vi "nanocal -- nuclear schottky fit V8.vi"() -> ()   [LabVIEW 2021] (continued)
\"Reoff\" -> 0.000000000000   ,  \"Imoff\" -> 0.000000000000   ,  \"στ1\" -> 0.000000000000   ,  \"στS\" -> 0.000000000000   ,  \"στN\" -> 0.000000000000   ,  \"τ11 \" -> 0.000000000000   ,  \"τ12\" -> 0.000000000000   ,  \"τ22\" -> 0.000000000000   ,  \"τN1\" -> 0.000000000000   ,  \"τN2\" -> 0.000000000000   ,  \"σηlogτ1 \" -> 0.000000000000   ,  \"σηlogτS\" -> 0.000000000000   ,  \"σηlogτN\" -> 0.000000000000   ,  \"σlogτ1\" -> 0.000000000000   ,  \"σlogτS\" -> 0.000000000000   ,  \"σlogτN\" -> 0.000000000000   ,  \"σητ1\" -> 0.000000000000   ,  \"σητS \" -> 0.000000000000   ,  \"σητN\" -> 0.000000000000    |>   , \n\"IDS0616_220610_RAW_cal__ref_\" ->   <|    \"ζ\" -> 0.021580744060   ,  \"τ1\" -> 0.018863304594   ,  \"τS\" -> 0.006040479317   ,  \"τN\" -> 0.000001032935   ,  \"τC\" -> 0.001981910818   ,  \"κ0\" -> 0.000000054950   ,  \"mm1\" -> 0.000031813825   ,  \"mm2\" -> 0.008120137752   ,  \"mm3\" -> 0.018865156416   ,  \"T\" -> 5.700000000000   ,  \"B\" -> 5.000000000000   ,  \"θ\" -> 90.000000000000   ,  \"Reoff\" -> 0.000000000000   ,  \"Imoff\" -> 0.000000000000   ,  \"στ1\" -> 0.086753021410   ,  \"στS\" -> 0.000000692284   ,  \"στN\" -> 0.000003593763   ,  \"τ11 \" -> 0.000000000000   ,  \"τ12\" -> 0.000000000000   ,  \"τ22\" -> 0.000000000000   ,  \"τN1\" -> 0.000000000000   ,  \"τN2\" -> 0.000000000000   ,  \"σηlogτ1 \" -> 0.078147370775   ,  \"σηlogτS\" -> 0.000000144573   ,  \"σηlogτN\" -> 0.120525182848   ,  \"σlogτ1\" -> 4.599036238749   ,  \"σlogτS\" -> 0.000114607395   ,  \"σlogτN\" -> 3.479176616069   ,  \"σητ1\" -> 0.001474117658   ,  \"σητS \" -> 0.000000000873   ,  \"σητN\" -> 0.000000124495    |>   , \n\"IDS0616_220610_RAW_cal__sam_\" ->   <|    \"ζ\" -> 0.000000000000   ,  \"τ1\" -> 0.000000000000   ,  \"τS\" -> 0.000000000000   ,  \"τN\" -> 0.000000000000   ,  \"τC\" -> 0.000000000000   ,  \"κ0\" -> 0.000000000000   ,  \"mm1\" -> 0.000000000000   ,  \"mm2\" -> 0.000000000000   ,  \"mm3\" -> 0.000000000000   ,  \"T\" -> 5.700000000000   ,  \"B\" -> 5.000000000000   ,  \"θ\" -> 90.000000000000   ,  \"Reoff\" -> 0.000000000000   ,  \"Imoff\" -> 0.000000000000   ,  \"στ1\" -> 0.000000000000   ,  \"στS\" -> 0.000000000000   ,  \"στN\" -> 0.000000000000   ,  \"τ11 \" -> 0.000000000000   ,  \"τ12\" -> 0.000000000000   ,  \"τ22\" -> 0.000000000000   ,  \"τN1\" -> 0.000000000000   ,  \"τN2\" -> 0.000000000000   ,  \"σηlogτ1 \" -> 0.000000000000   ,  \"σηlogτS\" -> 0.000000000000   ,  \"σηlogτN\" -> 0.000000000000   ,  \"σlogτ1\" -> 0.000000000000   ,  \"σlogτS\" -> 0.000000000000   ,  \"σlogτN\" -> 0.000000000000   ,  \"σητ1\" -> 0.000000000000   ,  \"σητS \" -> 0.000000000000   ,  \"σητN\" -> 0.000000000000    |>   , \n\"IDS0618_220610_RAW_cal__ref_\" ->   <|    \"ζ\" -> 0.037056549880   ,  \"τ1\" -> 0.018725402068   ,  \"τS\" -> 0.027332501190   ,  \"τN\" -> 0.000869050800   ,  \"τC\" -> 0.001924166709   ,  \"κ0\" -> 0.000000003749   ,  \"mm1\" -> 0.000064521634   ,  \"mm2\" -> 0.017486567655   ,  \"mm3\" -> 0.032345083697   ,  \"T\" -> 0.620000000000   ,  \"B\" -> 8.000000000000   ,  \"θ\" -> 90.000000000000   ,  \"Reoff\" -> 0.000000000000   ,  \"Imoff\" -> 0.000000000000   ,  \"στ1\" -> 0.000271617546   ,  \"στS\" -> 0.000004778676   ,  \"στN\" -> 0.000006417045   ,  \"τ11 \" -> 0.000000000000   ,  \"τ12\" -> 0.000000000000   ,  \"τ22\" -> 0.000000000000   ,  \"τN1\" -> 0.000000000000   ,  \"τN2\" -> 0.000000000000   ,  \"σηlogτ1 \" -> 0.143200048871   ,  \"σηlogτS\" -> 0.000251046394   ,  \"σηlogτN\" -> 0.135387426751   ,  \"σlogτ1\" -> 0.014505298451   ,  \"σlogτS\" -> 0.000174834918   ,  \"σlogτN\" -> 0.007383969732   ,  \"σητ1\" -> 0.002681478491   ,  \"σητS \" -> 0.000006861726   ,  \"σητN\" -> 0.000117658552    |>   , \n\"IDS0618_220610_RAW_cal__sam_\" ->   <|    \"ζ\" -> 0.000000000000   ,  \"τ1\" -> 0.000000000000   ,  \"τS\" -> 0.000000000000   ,  \"τN\" -> 0.000000000000   ,  \"τC\" -> 0.000000000000   ,  \"κ0\" -> 0.000000000000   ,  \"mm1\" -> 0.000000000000   ,  \"mm2\" -> 0.000000000000   ,  \"mm3\" -> 0.000000000000   ,  \"T\" -> 0.620000000000   ,  \"B\" -> 8.000000000000   ,  \"θ\" -> 90.000000000000   ,  \"Reoff\" -> 0.000000000000   ,  \"Imoff\" -> 0.000000000000   ,  \"στ1\" -> 0.000000000000   ,  \"στS\" -> 0.000000000000   ,  \"στN\" -> 0.000000000000   ,  \"τ11 \" -> 0.000000000000   ,  \"τ12\" -> 0.000000000000   ,  \"τ22\" -> 0.000000000000   ,  \"τN1\" -> 0.000000000000   ,  \"τN2\" -> 0.000000000000   ,  \"σηlogτ1 \" -> 0.000000000000   ,  \"σηlogτS\" -> 0.000000000000   ,  \"σηlogτN\" -> 0.000000000000   ,  \"σlogτ1\" -> 0.000000000000   ,  \"σlogτS\" -> 0.000000000000   ,  \"σlogτN\" -> 0.000000000000   ,  \"σητ1\" -> 0.000000000000   ,  \"σητS \" -> 0.000000000000   ,  \"σητN\" -> 0.000000000000    |>   , \n\"IDS0619_220610_RAW_cal__ref_\" ->   <|    \"ζ\" -> 0.022285334240   ,  \"τ1\" -> 0.023690071245   ,  \"τS\" -> 0.019354849977   ,  \"τN\" -> 0.000243089691   ,  \"τC\" -> 0.002524640152   ,  \"κ0\" -> 0.000000007189   ,  \"mm1\" -> 0.000048915318   ,  \"mm2\" -> 0.020603538471   ,  \"mm3\" -> 0.025596943911   ,  \"T\" -> 1.120000000000   ,  \"B\" -> 8.000000000000   ,  \"θ\" -> 90.000000000000   ,  \"Reoff\" -> 0.000000000000   ,  \"Imoff\" -> 0.000000000000   ,  \"στ1\" -> 0.000555160768   ,  \"στS\" -> 0.000001577745   ,  \"στN\" -> 0.000003357454   ,  \"τ11 \" -> 0.000000000000   ,  \"τ12\" -> 0.000000000000   ,  \"τ22\" -> 0.000000000000   ,  \"τN1\" -> 0.000000000000   ,  \"τN2\" -> 0.000000000000   ,  \"σηlogτ1 \" -> 0.107205120132   ,  \"σηlogτS\" -> 0.000041987587   ,  \"σηlogτN\" -> 0.127923521319   ,  \"σlogτ1\" -> 0.023434322442   ,  \"σlogτS\" -> 0.000081516797   ,  \"σlogτN\" -> 0.013811587104   ,  \"σητ1\" -> 0.002539696934   ,  \"σητS \" -> 0.000000812663   ,  \"σητN\" -> 0.000031096889    |>   , \n\"IDS0619_220610_RAW_cal__sam_\" ->   <|    \"ζ\" -> 0.000000000000   ,  \"τ1\" -> 0.000000000000   ,  \"τS\" -> 0.000000000000   ,  \"τN\" -> 0.000000000000   ,  \"τC\" -> 0.000000000000   ,  \"κ0\" -> 0.000000000000   ,  \"mm1\" -> 0.000000000000   ,  \"mm2\" -> 0.000000000000   ,  \"mm3\" -> 0.000000000000   ,  \"T\" -> 1.120000000000   ,  \"B\" -> 8.000000000000   ,  \"θ\" -> 90.000000000000   ,  \"Reoff\" -> 0.000000000000   ,  \"Imoff\" -> 0.000000000000   ,  \"στ1\" -> 0.000000000000   ,  \"στS\" -> 0.000000000000   ,  \"στN\" -> 0.000000000000   ,  \"τ11 \" -> 0.000000000000   ,  \"τ12\" -> 0.000000000000   ,  \"τ22\" -> 0.000000000000   ,  \"τN1\" -> 0.000000000000   ,  \"τN2\" -> 0.000000000000   ,  \"σηlogτ1 \" -> 0.000000000000   ,  \"σηlogτS\" -> 0.000000000000   ,  \"σηlogτN\" -> 0.000000000000   ,  \"σlogτ1\" -> 0.000000000000   ,  \"σlogτS\" -> 0.000000000000   ,  \"σlogτN\" -> 0.000000000000   ,  \"σητ1\" -> 0.000000000000   ,  \"σητS \" -> 0.000000000000   ,  \"σητN\" -> 0.000000000000    |>   , \n\"IDS0620_220610_RAW_cal__ref_\" ->   <|    \"ζ\" -> 0.017708509932   ,  \"τ1\" -> 0.018998736540   ,  \"τS\" -> 0.013522892780   ,  \"τN\" -> 0.000028025441   ,  \"τC\" -> 0.002986591079   ,  \"κ0\" -> 0.000000012545   ,  \"mm1\" -> 0.000042810551   ,  \"mm2\" -> 0.016516471437   ,  \"mm3\" -> 0.019216930422   ,  \"T\" -> 1.900000000000   ,  \"B\" -> 8.000000000000   ,  \"θ\" -> 90.000000000000   ,  \"Reoff\" -> -322448.979591836221   ,  \"Imoff\" -> 0.000000000000   ,  \"στ1\" -> 0.140264404305   ,  \"στS\" -> 0.000129912637   ,  \"στN\" -> 0.061579435163   ,  \"τ11 \" -> 0.000000000000   ,  \"τ12\" -> 0.000000000000   ,  \"τ22\" -> 0.000000000000   ,  \"τN1\" -> 0.000000000000   ,  \"τN2\" -> 0.000000000000   ,  \"σηlogτ1 \" -> 0.000000000000   ,  \"σηlogτS\" -> 0.000000000000   ,  \"σηlogτN\" -> 0.000000000000   ,  \"σlogτ1\" -> 0.000000000000   ,  \"σlogτS\" -> 0.000000000000   ,  \"σlogτN\" -> 0.000000000000   ,  \"σητ1\" -> 0.000000000000   ,  \"σητS \" -> 0.000000000000   ,  \"σητN\" -> 0.000000000000    |>   , \n\"IDS0620_220610_RAW_cal__sam_\" ->   <|    \"ζ\" -> 0.000000000000   ,  \"τ1\" -> 0.000000000000   ,  \"τS\" -> 0.000000000000   ,  \"τN\" -> 0.000000000000   ,  \"τC\" -> 0.000000000000   ,  \"κ0\" -> 0.000000000000   ,  \"mm1\" -> 0.000000000000   ,  \"mm2\" -> 0.000000000000   ,  \"mm3\" -> 0.000000000000   ,  \"T\" -> 1.900000000000   ,  \"B\" -> 8.000000000000   ,  \"θ\" -> 90.000000000000   ,  \"Reoff\" -> 0.000000000000   ,  \"Imoff\" -> 0.000000000000   ,  \"στ1\" -> 0.000000000000   ,  \"στS\" -> 0.000000000000   ,  \"στN\" -> 0.000000000000   ,  \"τ11 \" -> 0.000000000000   ,  \"τ12\" -> 0.000000000000   ,  \"τ22\" -> 0.000000000000   ,  \"τN1\" -> 0.000000000000   ,  \"τN2\" -> 0.000000000000   ,  \"σηlogτ1 \" -> 0.000000000000   ,  \"σηlogτS\" -> 0.000000000000   ,  \"σηlogτN\" -> 0.000000000000   ,  \"σlogτ1\" -> 0.000000000000   ,  \"σlogτS\" -> 0.000000000000   ,  \"σlogτN\" -> 0.000000000000   ,  \"σητ1\" -> 0.000000000000   ,  \"σητS \" -> 0.000000000000   ,  \"σητN\" -> 0.000000000000    |>   , \n\"IDS0621_220610_RAW_cal__ref_\" ->   <|    \"ζ\" -> 0.017222795450   ,  \"τ1\" -> 0.018997433498   ,  \"τS\" -> 0.009525458339   ,  \"τN\" -> 0.000004659714   ,  \"τC\" -> 0.002829107724   ,  \"κ0\" -> 0.000000022378   ,  \"mm1\" -> 0.000037185565   ,  \"mm2\" -> 0.012472383052   ,  \"mm3\" -> 0.019011225932   ,  \"T\" -> 3.100000000000   ,  \"B\" -> 8.000000000000   ,  \"θ\" -> 90.000000000000   ,  \"Reoff\" -> -175510.204081632662   ,  \"Imoff\" -> 0.000000000000   ,  \"στ1\" -> 1.184463822187   ,  \"στS\" -> 0.000211196697   ,  \"στN\" -> 0.576926670035   ,  \"τ11 \" -> 0.000000000000   ,  \"τ12\" -> 0.000000000000   ,  \"τ22\" -> 0.000000000000   ,  \"τN1\" -> 0.000000000000   ,  \"τN2\" -> 0.000000000000   ,  \"σηlogτ1 \" -> 0.000000000000   ,  \"σηlogτS\" -> 0.000000000000   ,  \"σηlogτN\" -> 0.000000000000   ,  \"σlogτ1\" -> 0.000000000000   ,  \"σlogτS\" -> 0.000000000000   ,  \"σlogτN\" -> 0.000000000000   ,  \"σητ1\" -> 0.000000000000   ,  \"σητS \" -> 0.000000000000   ,  \"σητN\" -> 0.000000000000    |>   , \n\"IDS0621_220610_RAW_cal__sam_\" ->   <|    \"ζ\" -> 0.000000000000   ,  \"τ1\" -> 0.000000000000   ,  \"τS\" -> 0.000000000000   ,  \"τN\" -> 0.000000000000   ,  \"τC\" -> 0.000000000000   ,  \"κ0\" -> 0.000000000000   ,  \"mm1\" -> 0.000000000000   ,  \"mm2\" -> 0.000000000000   ,  \"mm3\" -> 0.000000000000   ,  \"T\" -> 3.100000000000   ,  \"B\" -> 8.000000000000   ,  \"θ\" -> 90.000000000000   ,  \"Reoff\" -> 0.000000000000   ,  \"Imoff\" -> 0.000000000000   ,  \"στ1\" -> 0.000000000000   ,  \"στS\" -> 0.000000000000   ,  \"στN\" -> 0.000000000000   ,  \"τ11 \" -> 0.000000000000   ,  \"τ12\" -> 0.000000000000   ,  \"τ22\" -> 0.000000000000   ,  \"τN1\" -> 0.000000000000   ,  \"τN2\" -> 0.000000000000   ,  \"σηlogτ1 \" -> 0.000000000000   ,  \"σηlogτS\" -> 0.000000000000   ,  \"σηlogτN\" -> 0.000000000000   ,  \"σlogτ1\" -> 0.000000000000   ,  \"σlogτS\" -> 0.000000000000   ,  \"σlogτN\" -> 0.000000000000   ,  \"σητ1\" -> 0.000000000000   ,  \"σητS \" -> 0.000000000000   ,  \"σητN\" -> 0.000000000000    |>   , \n\"IDS0622_220610_RAW_cal__ref_\" ->   <|    \"ζ\" -> 0.018802685442   ,  \"τ1\" -> 0.018950322094   ,  \"τS\" -> 0.005932159284   ,  \"τN\" -> 0.000000659524   ,  \"τC\" -> 0.002206206702   ,  \"κ0\" -> 0.000000055128   ,  \"mm1\" -> 0.000029937026   ,  \"mm2\" -> 0.008219455491   ,  \"mm3\" -> 0.018951508013   ,  \"T\" -> 5.700000000000   ,  \"B\" -> 8.000000000000   ,  \"θ\" -> 90.000000000000   ,  \"Reoff\" -> -102040.816326530650   ,  \"Imoff\" -> 0.000000000000   ,  \"στ1\" -> 16.146666898973   ,  \"στS\" -> 0.000465319371   ,  \"στN\" -> 9.721658755114   ,  \"τ11 \" -> 0.000000000000   ,  \"τ12\" -> 0.000000000000   ,  \"τ22\" -> 0.000000000000   ,  \"τN1\" -> 0.000000000000   ,  \"τN2\" -> 0.000000000000   ,  \"σηlogτ1 \" -> 0.000000000000   ,  \"σηlogτS\" -> 0.000000000000   ,  \"σηlogτN\" -> 0.000000000000   ,  \"σlogτ1\" -> 0.000000000000   ,  \"σlogτS\" -> 0.000000000000   ,  \"σlogτN\" -> 0.000000000000   ,  \"σητ1\" -> 0.000000000000   ,  \"σητS \" -> 0.000000000000   ,  \"σητN\" -> 0.000000000000    |>   , \n\"IDS0622_220610_RAW_cal__sam_\" ->   <|    \"ζ\" -> 0.000000000000   ,  \"τ1\" -> 0.000000000000   ,  \"τS\" -> 0.000000000000   ,  \"τN\" -> 0.000000000000   ,  \"τC\" -> 0.000000000000   ,  \"κ0\" -> 0.000000000000   ,  \"mm1\" -> 0.000000000000   ,  \"mm2\" -> 0.000000000000   ,  \"mm3\" -> 0.000000000000   ,  \"T\" -> 5.700000000000   ,  \"B\" -> 8.000000000000   ,  \"θ\" -> 90.000000000000   ,  \"Reoff\" -> 0.000000000000   ,  \"Imoff\" -> 0.000000000000   ,  \"στ1\" -> 0.000000000000   ,  \"στS\" -> 0.000000000000   ,  \"στN\" -> 0.000000000000   ,  \"τ11 \" -> 0.000000000000   ,  \"τ12\" -> 0.000000000000   ,  \"τ22\" -> 0.000000000000   ,  \"τN1\" -> 0.000000000000   ,  \"τN2\" -> 0.000000000000   ,  \"σηlogτ1 \" -> 0.000000000000   ,  \"σηlogτS\" -> 0.000000000000   ,  \"σηlogτN\" -> 0.000000000000   ,  \"σlogτ1\" -> 0.000000000000   ,  \"σlogτS\" -> 0.000000000000   ,  \"σlogτN\" -> 0.000000000000   ,  \"σητ1\" -> 0.000000000000   ,  \"σητS \" -> 0.000000000000   ,  \"σητN\" -> 0.000000000000    |>   , \n\"IDS0624_220611_RAW_cal__ref_\" ->   <|    \"ζ\" -> 0.236945855383   ,  \"τ1\" -> 0.047928938722   ,  \"τS\" -> 0.040227228605   ,  \"τN\" -> 0.063271724608   ,  \"τC\" -> 0.000912127152   ,  \"κ0\" -> 0.000000000938   ,  \"mm1\" -> 0.000172149820   ,  \"mm2\" -> 0.014967198661   ,  \"mm3\" -> 0.161724318607   ,  \"T\" -> 0.200000000000   ,  \"B\" -> 10.000000000000   ,  \"θ\" -> 90.000000000000   ,  \"Reoff\" -> 0.000000000000   ,  \"Imoff\" -> 0.000000000000   ,  \"στ1\" -> 0.000044813488   ,  \"στS\" -> 0.000011433304   ,  \"στN\" -> 0.000038242973   ,  \"τ11 \" -> 0.000000000000   ,  \"τ12\" -> 0.000000000000   ,  \"τ22\" -> 0.000000000000   ,  \"τN1\" -> 0.000000000000   ,  \"τN2\" -> 0.000000000000   ,  \"σηlogτ1 \" -> 0.116274669687   ,  \"σηlogτS\" -> 0.004088772446   ,  \"σηlogτN\" -> 0.139680235023   ,  \"σlogτ1\" -> 0.000934998552   ,  \"σlogτS\" -> 0.000284218031   ,  \"σlogτN\" -> 0.000604424386   ,  \"σητ1\" -> 0.005572921518   ,  \"σητS \" -> 0.000164479984   ,  \"σητN\" -> 0.008837809363    |>   , \n\"IDS0624_220611_RAW_cal__sam_\" ->   <|    \"ζ\" -> 0.000000000000   ,  \"τ1\" -> 0.000000000000   ,  \"τS\" -> 0.000000000000   ,  \"τN\" -> 0.000000000000   ,  \"τC\" -> 0.000000000000   ,  \"κ0\" -> 0.000000000000   ,  \"mm1\" -> 0.000000000000   ,  \"mm2\" -> 0.000000000000   ,  \"mm3\" -> 0.000000000000   ,  \"T\" -> 0.200000000000   ,  \"B\" -> 10.000000000000   ,  \"θ\" -> 90.000000000000   ,  \"Reoff\" -> 0.000000000000   ,  \"Imoff\" -> 0.000000000000   ,  \"στ1\" -> 0.000000000000   ,  \"στS\" -> 0.000000000000   ,  \"στN\" -> 0.000000000000   ,  \"τ11 \" -> 0.000000000000   ,  \"τ12\" -> 0.000000000000   ,  \"τ22\" -> 0.000000000000   ,  \"τN1\" -> 0.000000000000   ,  \"τN2\" -> 0.000000000000   ,  \"σηlogτ1 \" -> 0.000000000000   ,  \"σηlogτS\" -> 0.000000000000   ,  \"σηlogτN\" -> 0.000000000000   ,  \"σlogτ1\" -> 0.000000000000   ,  \"σlogτS\" -> 0.000000000000   ,  \"σlogτN\" -> 0.000000000000   ,  \"σητ1\" -> 0.000000000000   ,  \"σητS \" -> 0.000000000000   ,  \"σητN\" -> 0.000000000000    |>   , \n\"IDS0625_220611_RAW_cal__ref_\" ->   <|    \"ζ\" -> 0.327025562837   ,  \"τ1\" -> 0.059339000703   ,  \"τS\" -> 0.049734125673   ,  \"τN\" -> 0.113807285584   ,  \"τC\" -> 0.000851803177   ,  \"κ0\" -> 0.000000000764   ,  \"mm1\" -> 0.000207869539   ,  \"mm2\" -> 0.015100054741   ,  \"mm3\" -> 0.261906512920   ,  \"T\" -> 0.170000000000   ,  \"B\" -> 10.000000000000   ,  \"θ\" -> 90.000000000000   ,  \"Reoff\" -> 0.000000000000   ,  \"Imoff\" -> 0.000000000000   ,  \"στ1\" -> 0.000104711962   ,  \"στS\" -> 0.000034023066   ,  \"στN\" -> 0.000130609835   ,  \"τ11 \" -> 0.000000000000   ,  \"τ12\" -> 0.000000000000   ,  \"τ22\" -> 0.000000000000   ,  \"τN1\" -> 0.000000000000   ,  \"τN2\" -> 0.000000000000   ,  \"σηlogτ1 \" -> 0.122338501744   ,  \"σηlogτS\" -> 0.005402997656   ,  \"σηlogτN\" -> 0.146638117575   ,  \"σlogτ1\" -> 0.001764639795   ,  \"σlogτS\" -> 0.000684099005   ,  \"σlogτN\" -> 0.001147640370   ,  \"σητ1\" -> 0.007259444441   ,  \"σητS \" -> 0.000268713364   ,  \"σητN\" -> 0.016688486124    |>   , \n\"IDS0625_220611_RAW_cal__sam_\" ->   <|    \"ζ\" -> 0.000000000000   ,  \"τ1\" -> 0.000000000000   ,  \"τS\" -> 0.000000000000   ,  \"τN\" -> 0.000000000000   ,  \"τC\" -> 0.000000000000   ,  \"κ0\" -> 0.000000000000   ,  \"mm1\" -> 0.000000000000   ,  \"mm2\" -> 0.000000000000   ,  \"mm3\" -> 0.000000000000   ,  \"T\" -> 0.170000000000   ,  \"B\" -> 10.000000000000   ,  \"θ\" -> 90.000000000000   ,  \"Reoff\" -> 0.000000000000   ,  \"Imoff\" -> 0.000000000000   ,  \"στ1\" -> 0.000000000000   ,  \"στS\" -> 0.000000000000   ,  \"στN\" -> 0.000000000000   ,  \"τ11 \" -> 0.000000000000   ,  \"τ12\" -> 0.000000000000   ,  \"τ22\" -> 0.000000000000   ,  \"τN1\" -> 0.000000000000   ,  \"τN2\" -> 0.000000000000   ,  \"σηlogτ1 \" -> 0.000000000000   ,  \"σηlogτS\" -> 0.000000000000   ,  \"σηlogτN\" -> 0.000000000000   ,  \"σlogτ1\" -> 0.000000000000   ,  \"σlogτS\" -> 0.000000000000   ,  \"σlogτN\" -> 0.000000000000   ,  \"σητ1\" -> 0.000000000000   ,  \"σητS \" -> 0.000000000000   ,  \"σητN\" -> 0.000000000000    |>   , \n\"IDS0626_220611_RAW_cal__ref_\" ->   <|    \"ζ\" -> 0.413398104897   ,  \"τ1\" -> 0.067875745841   ,  \"τS\" -> 0.063032069928   ,  \"τN\" -> 0.190750500145   ,  \"τC\" -> 0.000838943281   ,  \"κ0\" -> 0.000000000639   ,  \"mm1\" -> 0.000243732197   ,  \"mm2\" -> 0.014761841095   ,  \"mm3\" -> 0.412404919429   ,  \"T\" -> 0.150000000000   ,  \"B\" -> 10.000000000000   ,  \"θ\" -> 90.000000000000   ,  \"Reoff\" -> 0.000000000000   ,  \"Imoff\" -> 0.000000000000   ,  \"στ1\" -> 0.000192212133   ,  \"στS\" -> 0.000084399120   ,  \"στN\" -> 0.000341477666   ,  \"τ11 \" -> 0.000000000000   ,  \"τ12\" -> 0.000000000000   ,  \"τ22\" -> 0.000000000000   ,  \"τN1\" -> 0.000000000000   ,  \"τN2\" -> 0.000000000000   ,  \"σηlogτ1 \" -> 0.134243827848   ,  \"σηlogτS\" -> 0.007146311807   ,  \"σηlogτN\" -> 0.157301214691   ,  \"σlogτ1\" -> 0.002831823508   ,  \"σlogτS\" -> 0.001338986966   ,  \"σlogτN\" -> 0.001790179662   ,  \"σητ1\" -> 0.009111899940   ,  \"σητS \" -> 0.000450446826   ,  \"σητN\" -> 0.030005285376    |>   , \n\"IDS0626_220611_RAW_cal__sam_\" ->   <|    \"ζ\" -> 0.000000000000   ,  \"τ1\" -> 0.000000000000   ,  \"τS\" -> 0.000000000000   ,  \"τN\" -> 0.000000000000   ,  \"τC\" -> 0.000000000000   ,  \"κ0\" -> 0.000000000000   ,  \"mm1\" -> 0.000000000000   ,  \"mm2\" -> 0.000000000000   ,  \"mm3\" -> 0.000000000000   ,  \"T\" -> 0.150000000000   ,  \"B\" -> 10.000000000000   ,  \"θ\" -> 90.000000000000   ,  \"Reoff\" -> 0.000000000000   ,  \"Imoff\" -> 0.000000000000   ,  \"στ1\" -> 0.000000000000   ,  \"στS\" -> 0.000000000000   ,  \"στN\" -> 0.000000000000   ,  \"τ11 \" -> 0.000000000000   ,  \"τ12\" -> 0.000000000000   ,  \"τ22\" -> 0.000000000000   ,  \"τN1\" -> 0.000000000000   ,  \"τN2\" -> 0.000000000000   ,  \"σηlogτ1 \" -> 0.000000000000   ,  \"σηlogτS\" -> 0.000000000000   ,  \"σηlogτN\" -> 0.000000000000   ,  \"σlogτ1\" -> 0.000000000000   ,  \"σlogτS\" -> 0.000000000000   ,  \"σlogτN\" -> 0.000000000000   ,  \"σητ1\" -> 0.000000000000   ,  \"σητS \" -> 0.000000000000   ,  \"σητN\" -> 0.000000000000    |>   , \n\"IDS0627_220611_RAW_cal__ref_\" ->   <|    \"ζ\" -> 0.627345868591   ,  \"τ1\" -> 0.082512030624   ,  \"τS\" -> 0.111539942988   ,  \"τN\" -> 0.459820261039   ,  \"τC\" -> 0.000856922343   ,  \"κ0\" -> 0.000000000480   ,  \"mm1\" -> 0.000329372323   ,  \"mm2\" -> 0.015054692399   ,  \"mm3\" -> 0.997785555745   ,  \"T\" -> 0.120000000000   ,  \"B\" -> 10.000000000000   ,  \"θ\" -> 90.000000000000   ,  \"Reoff\" -> 0.000000000000   ,  \"Imoff\" -> 0.000000000000   ,  \"στ1\" -> 0.000378111787   ,  \"στS\" -> 0.000316880051   ,  \"στN\" -> 0.001160403216   ,  \"τ11 \" -> 0.000000000000   ,  \"τ12\" -> 0.000000000000   ,  \"τ22\" -> 0.000000000000   ,  \"τN1\" -> 0.000000000000   ,  \"τN2\" -> 0.000000000000   ,  \"σηlogτ1 \" -> 0.166706810062   ,  \"σηlogτS\" -> 0.011257222829   ,  \"σηlogτN\" -> 0.184131010310   ,  \"σlogτ1\" -> 0.004582504926   ,  \"σlogτS\" -> 0.002840955825   ,  \"σlogτN\" -> 0.002523601752   ,  \"σητ1\" -> 0.013755317417   ,  \"σητS \" -> 0.001255629993   ,  \"σητN\" -> 0.084667169226    |>   , \n\"IDS0627_220611_RAW_cal__sam_\" ->   <|    \"ζ\" -> 0.000000000000   ,  \"τ1\" -> 0.000000000000   ,  \"τS\" -> 0.000000000000   ,  \"τN\" -> 0.000000000000   ,  \"τC\" -> 0.000000000000   ,  \"κ0\" -> 0.000000000000   ,  \"mm1\" -> 0.000000000000   ,  \"mm2\" -> 0.000000000000   ,  \"mm3\" -> 0.000000000000   ,  \"T\" -> 0.120000000000   ,  \"B\" -> 10.000000000000   ,  \"θ\" -> 90.000000000000   ,  \"Reoff\" -> 0.000000000000   ,  \"Imoff\" -> 0.000000000000   ,  \"στ1\" -> 0.000000000000   ,  \"στS\" -> 0.000000000000   ,  \"στN\" -> 0.000000000000   ,  \"τ11 \" -> 0.000000000000   ,  \"τ12\" -> 0.000000000000   ,  \"τ22\" -> 0.000000000000   ,  \"τN1\" -> 0.000000000000   ,  \"τN2\" -> 0.000000000000   ,  \"σηlogτ1 \" -> 0.000000000000   ,  \"σηlogτS\" -> 0.000000000000   ,  \"σηlogτN\" -> 0.000000000000   ,  \"σlogτ1\" -> 0.000000000000   ,  \"σlogτS\" -> 0.000000000000   ,  \"σlogτN\" -> 0.000000000000   ,  \"σητ1\" -> 0.000000000000   ,  \"σητS \" -> 0.000000000000   ,  \"σητN\" -> 0.000000000000    |>   , \n\"IDS0628_220611_RAW_cal__ref_\" ->   <|    \"ζ\" -> 0.152770220737   ,  \"τ1\" -> 0.036198364925   ,  \"τS\" -> 0.033549808091   ,  \"τN\" -> 0.027206802922   ,  \"τC\" -> 0.001036197063   ,  \"κ0\" -> 0.000000001265   ,  \"mm1\" -> 0.000134182447   ,  \"mm2\" -> 0.015662270095   ,  \"mm3\" -> 0.091476521334   ,  \"T\" -> 0.250000000000   ,  \"B\" -> 10.000000000000   ,  \"θ\" -> 90.000000000000   ,  \"Reoff\" -> 0.000000000000   ,  \"Imoff\" -> 0.000000000000   ,  \"στ1\" -> 0.000013390131   ,  \"στS\" -> 0.000002421606   ,  \"στN\" -> 0.000006177026   ,  \"τ11 \" -> 0.000000000000   ,  \"τ12\" -> 0.000000000000   ,  \"τ22\" -> 0.000000000000   ,  \"τN1\" -> 0.000000000000   ,  \"τN2\" -> 0.000000000000   ,  \"σηlogτ1 \" -> 0.116147333813   ,  \"σηlogτS\" -> 0.002721053400   ,  \"σηlogτN\" -> 0.134955883548   ,  \"σlogτ1\" -> 0.000369909834   ,  \"σlogτS\" -> 0.000072179437   ,  \"σlogτN\" -> 0.000227039759   ,  \"σητ1\" -> 0.004204343574   ,  \"σητS \" -> 0.000091290819   ,  \"σητN\" -> 0.003671718127    |>   , \n\"IDS0628_220611_RAW_cal__sam_\" ->   <|    \"ζ\" -> 0.000000000000   ,  \"τ1\" -> 0.000000000000   ,  \"τS\" -> 0.000000000000   ,  \"τN\" -> 0.000000000000   ,  \"τC\" -> 0.000000000000   ,  \"κ0\" -> 0.000000000000   ,  \"mm1\" -> 0.000000000000   ,  \"mm2\" -> 0.000000000000   ,  \"mm3\" -> 0.000000000000   ,  \"T\" -> 0.250000000000   ,  \"B\" -> 10.000000000000   ,  \"θ\" -> 90.000000000000   ,  \"Reoff\" -> 0.000000000000   ,  \"Imoff\" -> 0.000000000000   ,  \"στ1\" -> 0.000000000000   ,  \"στS\" -> 0.000000000000   ,  \"στN\" -> 0.000000000000   ,  \"τ11 \" -> 0.000000000000   ,  \"τ12\" -> 0.000000000000   ,  \"τ22\" -> 0.000000000000   ,  \"τN1\" -> 0.000000000000   ,  \"τN2\" -> 0.000000000000   ,  \"σηlogτ1 \" -> 0.000000000000   ,  \"σηlogτS\" -> 0.000000000000   ,  \"σηlogτN\" -> 0.000000000000   ,  \"σlogτ1\" -> 0.000000000000   ,  \"σlogτS\" -> 0.000000000000   ,  \"σlogτN\" -> 0.000000000000   ,  \"σητ1\" -> 0.000000000000   ,  \"σητS \" -> 0.000000000000   ,  \"σητN\" -> 0.000000000000    |>   , \n\"IDS0629_220611_RAW_cal__ref_\" ->   <|    \"ζ\" -> 0.104961058193   ,  \"τ1\" -> 0.030489437824   ,  \"τS\" -> 0.030011872176   ,  \"τN\" -> 0.014021025099   ,  \"τC\" -> 0.001158647608   ,  \"κ0\" -> 0.000000001606   ,  \"mm1\" -> 0.000106671353   ,  \"mm2\" -> 0.016335963882   ,  \"mm3\" -> 0.063860086966   ,  \"T\" -> 0.300000000000   ,  \"B\" -> 10.000000000000   ,  \"θ\" -> 90.000000000000   ,  \"Reoff\" -> 0.000000000000   ,  \"Imoff\" -> 0.000000000000   ,  \"στ1\" -> 0.000007085631   ,  \"στS\" -> 0.000000880275   ,  \"στN\" -> 0.000001925171   ,  \"τ11 \" -> 0.000000000000   ,  \"τ12\" -> 0.000000000000   ,  \"τ22\" -> 0.000000000000   ,  \"τN1\" -> 0.000000000000   ,  \"τN2\" -> 0.000000000000   ,  \"σηlogτ1 \" -> 0.117123612292   ,  \"σηlogτS\" -> 0.001807335056   ,  \"σηlogτN\" -> 0.132991316128   ,  \"σlogτ1\" -> 0.000232396245   ,  \"σlogτS\" -> 0.000029330901   ,  \"σlogτN\" -> 0.000137306042   ,  \"σητ1\" -> 0.003571033095   ,  \"σητS \" -> 0.000054241509   ,  \"σητN\" -> 0.001864674581    |>   , \n\"IDS0629_220611_RAW_cal__sam_\" ->   <|    \"ζ\" -> 0.000000000000   ,  \"τ1\" -> 0.000000000000   ,  \"τS\" -> 0.000000000000   ,  \"τN\" -> 0.000000000000   ,  \"τC\" -> 0.000000000000   ,  \"κ0\" -> 0.000000000000   ,  \"mm1\" -> 0.000000000000   ,  \"mm2\" -> 0.000000000000   ,  \"mm3\" -> 0.000000000000   ,  \"T\" -> 0.300000000000   ,  \"B\" -> 10.000000000000   ,  \"θ\" -> 90.000000000000   ,  \"Reoff\" -> 0.000000000000   ,  \"Imoff\" -> 0.000000000000   ,  \"στ1\" -> 0.000000000000   ,  \"στS\" -> 0.000000000000   ,  \"στN\" -> 0.000000000000   ,  \"τ11 \" -> 0.000000000000   ,  \"τ12\" -> 0.000000000000   ,  \"τ22\" -> 0.000000000000   ,  \"τN1\" -> 0.000000000000   ,  \"τN2\" -> 0.000000000000   ,  \"σηlogτ1 \" -> 0.000000000000   ,  \"σηlogτS\" -> 0.000000000000   ,  \"σηlogτN\" -> 0.000000000000   ,  \"σlogτ1\" -> 0.000000000000   ,  \"σlogτS\" -> 0.000000000000   ,  \"σlogτN\" -> 0.000000000000   ,  \"σητ1\" -> 0.000000000000   ,  \"σητS \" -> 0.000000000000   ,  \"σητN\" -> 0.000000000000    |>   , \n\"IDS0630_220611_RAW_cal__ref_\" ->   <|    \"ζ\" -> 0.075687079530   ,  \"τ1\" -> 0.025692917456   ,  \"τS\" -> 0.027518005635   ,  \"τN\" -> 0.007256477389   ,  \"τC\" -> 0.001413406836   ,  \"κ0\" -> 0.000000002017   ,  \"mm1\" -> 0.000095205662   ,  \"mm2\" -> 0.016621150095   ,  \"mm3\" -> 0.047796430621   ,  \"T\" -> 0.360000000000   ,  \"B\" -> 10.000000000000   ,  \"θ\" -> 90.000000000000   ,  \"Reoff\" -> 0.000000000000   ,  \"Imoff\" -> 0.000000000000   ,  \"στ1\" -> 0.000009211361   ,  \"στS\" -> 0.000000780336   ,  \"στN\" -> 0.000001470575   ,  \"τ11 \" -> 0.000000000000   ,  \"τ12\" -> 0.000000000000   ,  \"τ22\" -> 0.000000000000   ,  \"τN1\" -> 0.000000000000   ,  \"τN2\" -> 0.000000000000   ,  \"σηlogτ1 \" -> 0.121353390675   ,  \"σηlogτS\" -> 0.001216073528   ,  \"σηlogτN\" -> 0.132703139128   ,  \"σlogτ1\" -> 0.000358517508   ,  \"σlogτS\" -> 0.000028357288   ,  \"σlogτN\" -> 0.000202656857   ,  \"σητ1\" -> 0.003117922650   ,  \"σητS \" -> 0.000033463918   ,  \"σητN\" -> 0.000962957328    |>   , \n\"IDS0630_220611_RAW_cal__sam_\" ->   <|    \"ζ\" -> 0.000000000000   ,  \"τ1\" -> 0.000000000000   ,  \"τS\" -> 0.000000000000   ,  \"τN\" -> 0.000000000000   ,  \"τC\" -> 0.000000000000   ,  \"κ0\" -> 0.000000000000   ,  \"mm1\" -> 0.000000000000   ,  \"mm2\" -> 0.000000000000   ,  \"mm3\" -> 0.000000000000   ,  \"T\" -> 0.360000000000   ,  \"B\" -> 10.000000000000   ,  \"θ\" -> 90.000000000000   ,  \"Reoff\" -> 0.000000000000   ,  \"Imoff\" -> 0.000000000000   ,  \"στ1\" -> 0.000000000000   ,  \"στS\" -> 0.000000000000   ,  \"στN\" -> 0.000000000000   ,  \"τ11 \" -> 0.000000000000   ,  \"τ12\" -> 0.000000000000   ,  \"τ22\" -> 0.000000000000   ,  \"τN1\" -> 0.000000000000   ,  \"τN2\" -> 0.000000000000   ,  \"σηlogτ1 \" -> 0.000000000000   ,  \"σηlogτS\" -> 0.000000000000   ,  \"σηlogτN\" -> 0.000000000000   ,  \"σlogτ1\" -> 0.000000000000   ,  \"σlogτS\" -> 0.000000000000   ,  \"σlogτN\" -> 0.000000000000   ,  \"σητ1\" -> 0.000000000000   ,  \"σητS \" -> 0.000000000000   ,  \"σητN\" -> 0.000000000000    |>   , \n\"IDS0631_220611_RAW_cal__ref_\" ->   <|    \"ζ\" -> 0.058935240336   ,  \"τ1\" -> 0.021193518217   ,  \"τS\" -> 0.025799898485   ,  \"τN\" -> 0.004769009758   ,  \"τC\" -> 0.001612077295   ,  \"κ0\" -> 0.000000002413   ,  \"mm1\" -> 0.000084967559   ,  \"mm2\" -> 0.015406650386   ,  \"mm3\" -> 0.039684471766   ,  \"T\" -> 0.420000000000   ,  \"B\" -> 10.000000000000   ,  \"θ\" -> 90.000000000000   ,  \"Reoff\" -> 0.000000000000   ,  \"Imoff\" -> 0.000000000000   ,  \"στ1\" -> 0.000010740234   ,  \"στS\" -> 0.000000797297   ,  \"στN\" -> 0.000001307044   ,  \"τ11 \" -> 0.000000000000   ,  \"τ12\" -> 0.000000000000   ,  \"τ22\" -> 0.000000000000   ,  \"τN1\" -> 0.000000000000   ,  \"τN2\" -> 0.000000000000   ,  \"σηlogτ1 \" -> 0.129682628231   ,  \"σηlogτS\" -> 0.001061043633   ,  \"σηlogτN\" -> 0.134054055610   ,  \"σlogτ1\" -> 0.000506769772   ,  \"σlogτS\" -> 0.000030903120   ,  \"σlogτN\" -> 0.000274070212   ,  \"σητ1\" -> 0.002748431144   ,  \"σητS \" -> 0.000027374818   ,  \"σητN\" -> 0.000639305099    |>   , \n\"IDS0631_220611_RAW_cal__sam_\" ->   <|    \"ζ\" -> 0.000000000000   ,  \"τ1\" -> 0.000000000000   ,  \"τS\" -> 0.000000000000   ,  \"τN\" -> 0.000000000000   ,  \"τC\" -> 0.000000000000   ,  \"κ0\" -> 0.000000000000   ,  \"mm1\" -> 0.000000000000   ,  \"mm2\" -> 0.000000000000   ,  \"mm3\" -> 0.000000000000   ,  \"T\" -> 0.420000000000   ,  \"B\" -> 10.000000000000   ,  \"θ\" -> 90.000000000000   ,  \"Reoff\" -> 0.000000000000   ,  \"Imoff\" -> 0.000000000000   ,  \"στ1\" -> 0.000000000000   ,  \"στS\" -> 0.000000000000   ,  \"στN\" -> 0.000000000000   ,  \"τ11 \" -> 0.000000000000   ,  \"τ12\" -> 0.000000000000   ,  \"τ22\" -> 0.000000000000   ,  \"τN1\" -> 0.000000000000   ,  \"τN2\" -> 0.000000000000   ,  \"σηlogτ1 \" -> 0.000000000000   ,  \"σηlogτS\" -> 0.000000000000   ,  \"σηlogτN\" -> 0.000000000000   ,  \"σlogτ1\" -> 0.000000000000   ,  \"σlogτS\" -> 0.000000000000   ,  \"σlogτN\" -> 0.000000000000   ,  \"σητ1\" -> 0.000000000000   ,  \"σητS \" -> 0.000000000000   ,  \"σητN\" -> 0.000000000000    |>   , \n\"IDS0632_220611_RAW_cal__ref_\" ->   <|    \"ζ\" -> 0.044055217720   ,  \"τ1\" -> 0.018398673141   ,  \"τS\" -> 0.024296902753   ,  \"τN\" -> 0.002237219247   ,  \"τC\" -> 0.001705422897   ,  \"κ0\" -> 0.000000003103   ,  \"mm1\" -> 0.000067596634   ,  \"mm2\" -> 0.015331750365   ,  \"mm3\" -> 0.032407837560   ,  \"T\" -> 0.520000000000   ,  \"B\" -> 10.000000000000   ,  \"θ\" -> 90.000000000000   ,  \"Reoff\" -> 0.000000000000   ,  \"Imoff\" -> 0.000000000000   ,  \"στ1\" -> 0.000025900073   ,  \"στS\" -> 0.000001114973   ,  \"στN\" -> 0.000001649689   ,  \"τ11 \" -> 0.000000000000   ,  \"τ12\" -> 0.000000000000   ,  \"τ22\" -> 0.000000000000   ,  \"τN1\" -> 0.000000000000   ,  \"τN2\" -> 0.000000000000   ,  \"σηlogτ1 \" -> 0.135453082912   ,  \"σηlogτS\" -> 0.000614451179   ,  \"σηlogτN\" -> 0.134477904132   ,  \"σlogτ1\" -> 0.001407714152   ,  \"σlogτS\" -> 0.000045889504   ,  \"σlogτN\" -> 0.000737383723   ,  \"σητ1\" -> 0.002492156998   ,  \"σητS \" -> 0.000014929261   ,  \"σητN\" -> 0.000300856555    |>   , \n\"IDS0632_220611_RAW_cal__sam_\" ->   <|    \"ζ\" -> 0.000000000000   ,  \"τ1\" -> 0.000000000000   ,  \"τS\" -> 0.000000000000   ,  \"τN\" -> 0.000000000000   ,  \"τC\" -> 0.000000000000   ,  \"κ0\" -> 0.000000000000   ,  \"mm1\" -> 0.000000000000   ,  \"mm2\" -> 0.000000000000   ,  \"mm3\" -> 0.000000000000   ,  \"T\" -> 0.520000000000   ,  \"B\" -> 10.000000000000   ,  \"θ\" -> 90.000000000000   ,  \"Reoff\" -> 0.000000000000   ,  \"Imoff\" -> 0.000000000000   ,  \"στ1\" -> 0.000000000000   ,  \"στS\" -> 0.000000000000   ,  \"στN\" -> 0.000000000000   ,  \"τ11 \" -> 0.000000000000   ,  \"τ12\" -> 0.000000000000   ,  \"τ22\" -> 0.000000000000   ,  \"τN1\" -> 0.000000000000   ,  \"τN2\" -> 0.000000000000   ,  \"σηlogτ1 \" -> 0.000000000000   ,  \"σηlogτS\" -> 0.000000000000   ,  \"σηlogτN\" -> 0.000000000000   ,  \"σlogτ1\" -> 0.000000000000   ,  \"σlogτS\" -> 0.000000000000   ,  \"σlogτN\" -> 0.000000000000   ,  \"σητ1\" -> 0.000000000000   ,  \"σητS \" -> 0.000000000000   ,  \"σητN\" -> 0.000000000000    |>   , \n\"IDS0633_220611_RAW_cal__ref_\" ->   <|    \"ζ\" -> 0.034142201059   ,  \"τ1\" -> 0.016889163361   ,  \"τS\" -> 0.022852529077   ,  \"τN\" -> 0.001326577994   ,  \"τC\" -> 0.002278925943   ,  \"κ0\" -> 0.000000003798   ,  \"mm1\" -> 0.000068802803   ,  \"mm2\" -> 0.014993961538   ,  \"mm3\" -> 0.029109959969   ,  \"T\" -> 0.620000000000   ,  \"B\" -> 10.000000000000   ,  \"θ\" -> 90.000000000000   ,  \"Reoff\" -> 0.000000000000   ,  \"Imoff\" -> 0.000000000000   ,  \"στ1\" -> 0.000028192933   ,  \"στS\" -> 0.000000811322   ,  \"στN\" -> 0.000001142735   ,  \"τ11 \" -> 0.000000000000   ,  \"τ12\" -> 0.000000000000   ,  \"τ22\" -> 0.000000000000   ,  \"τN1\" -> 0.000000000000   ,  \"τN2\" -> 0.000000000000   ,  \"σηlogτ1 \" -> 0.138852812126   ,  \"σηlogτS\" -> 0.000419923481   ,  \"σηlogτN\" -> 0.134804184987   ,  \"σlogτ1\" -> 0.001669291277   ,  \"σlogτS\" -> 0.000035502510   ,  \"σlogτN\" -> 0.000861415426   ,  \"σητ1\" -> 0.002345107827   ,  \"σητS \" -> 0.000009596314   ,  \"σητN\" -> 0.000178828265    |>   , \n\"IDS0633_220611_RAW_cal__sam_\" ->   <|    \"ζ\" -> 0.000000000000   ,  \"τ1\" -> 0.000000000000   ,  \"τS\" -> 0.000000000000   ,  \"τN\" -> 0.000000000000   ,  \"τC\" -> 0.000000000000   ,  \"κ0\" -> 0.000000000000   ,  \"mm1\" -> 0.000000000000   ,  \"mm2\" -> 0.000000000000   ,  \"mm3\" -> 0.000000000000   ,  \"T\" -> 0.620000000000   ,  \"B\" -> 10.000000000000   ,  \"θ\" -> 90.000000000000   ,  \"Reoff\" -> 0.000000000000   ,  \"Imoff\" -> 0.000000000000   ,  \"στ1\" -> 0.000000000000   ,  \"στS\" -> 0.000000000000   ,  \"στN\" -> 0.000000000000   ,  \"τ11 \" -> 0.000000000000   ,  \"τ12\" -> 0.000000000000   ,  \"τ22\" -> 0.000000000000   ,  \"τN1\" -> 0.000000000000   ,  \"τN2\" -> 0.000000000000   ,  \"σηlogτ1 \" -> 0.000000000000   ,  \"σηlogτS\" -> 0.000000000000   ,  \"σηlogτN\" -> 0.000000000000   ,  \"σlogτ1\" -> 0.000000000000   ,  \"σlogτS\" -> 0.000000000000   ,  \"σlogτN\" -> 0.000000000000   ,  \"σητ1\" -> 0.000000000000   ,  \"σητS \" -> 0.000000000000   ,  \"σητN\" -> 0.000000000000    |>   , \n\"IDS0634_220612_RAW_cal__ref_\" ->   <|    \"ζ\" -> 0.026094794498   ,  \"τ1\" -> 0.017613964803   ,  \"τS\" -> 0.020608194694   ,  \"τN\" -> 0.000565779347   ,  \"τC\" -> 0.002821541401   ,  \"κ0\" -> 0.000000005177   ,  \"mm1\" -> 0.000063475218   ,  \"mm2\" -> 0.016356491351   ,  \"mm3\" -> 0.025742044178   ,  \"T\" -> 0.820000000000   ,  \"B\" -> 10.000000000000   ,  \"θ\" -> 90.000000000000   ,  \"Reoff\" -> 0.000000000000   ,  \"Imoff\" -> 0.000000000000   ,  \"στ1\" -> 0.000096609701   ,  \"στS\" -> 0.000001077026   ,  \"στN\" -> 0.000001637448   ,  \"τ11 \" -> 0.000000000000   ,  \"τ12\" -> 0.000000000000   ,  \"τ22\" -> 0.000000000000   ,  \"τN1\" -> 0.000000000000   ,  \"τN2\" -> 0.000000000000   ,  \"σηlogτ1 \" -> 0.129941381525   ,  \"σηlogτS\" -> 0.000167044779   ,  \"σηlogτN\" -> 0.132803601967   ,  \"σlogτ1\" -> 0.005484835568   ,  \"σlogτS\" -> 0.000052262034   ,  \"σlogτN\" -> 0.002894146508   ,  \"σητ1\" -> 0.002288782921   ,  \"σητS \" -> 0.000003442491   ,  \"σητN\" -> 0.000075137535    |>   , \n\"IDS0634_220612_RAW_cal__sam_\" ->   <|    \"ζ\" -> 0.000000000000   ,  \"τ1\" -> 0.000000000000   ,  \"τS\" -> 0.000000000000   ,  \"τN\" -> 0.000000000000   ,  \"τC\" -> 0.000000000000   ,  \"κ0\" -> 0.000000000000   ,  \"mm1\" -> 0.000000000000   ,  \"mm2\" -> 0.000000000000   ,  \"mm3\" -> 0.000000000000   ,  \"T\" -> 0.820000000000   ,  \"B\" -> 10.000000000000   ,  \"θ\" -> 90.000000000000   ,  \"Reoff\" -> 0.000000000000   ,  \"Imoff\" -> 0.000000000000   ,  \"στ1\" -> 0.000000000000   ,  \"στS\" -> 0.000000000000   ,  \"στN\" -> 0.000000000000   ,  \"τ11 \" -> 0.000000000000   ,  \"τ12\" -> 0.000000000000   ,  \"τ22\" -> 0.000000000000   ,  \"τN1\" -> 0.000000000000   ,  \"τN2\" -> 0.000000000000   ,  \"σηlogτ1 \" -> 0.000000000000   ,  \"σηlogτS\" -> 0.000000000000   ,  \"σηlogτN\" -> 0.000000000000   ,  \"σlogτ1\" -> 0.000000000000   ,  \"σlogτS\" -> 0.000000000000   ,  \"σlogτN\" -> 0.000000000000   ,  \"σητ1\" -> 0.000000000000   ,  \"σητS \" -> 0.000000000000   ,  \"σητN\" -> 0.000000000000    |>   , \n\"IDS0635_220612_RAW_cal__ref_\" ->   <|    \"ζ\" -> 0.022302849506   ,  \"τ1\" -> 0.019271147098   ,  \"τS\" -> 0.018127459113   ,  \"τN\" -> 0.000191566174   ,  \"τC\" -> 0.003097458701   ,  \"κ0\" -> 0.000000007267   ,  \"mm1\" -> 0.000058053364   ,  \"mm2\" -> 0.018210505048   ,  \"mm3\" -> 0.022827639139   ,  \"T\" -> 1.120000000000   ,  \"B\" -> 10.000000000000   ,  \"θ\" -> 90.000000000000   ,  \"Reoff\" -> 0.000000000000   ,  \"Imoff\" -> 0.000000000000   ,  \"στ1\" -> 0.000470741477   ,  \"στS\" -> 0.000001456602   ,  \"στN\" -> 0.000002601409   ,  \"τ11 \" -> 0.000000000000   ,  \"τ12\" -> 0.000000000000   ,  \"τ22\" -> 0.000000000000   ,  \"τN1\" -> 0.000000000000   ,  \"τN2\" -> 0.000000000000   ,  \"σηlogτ1 \" -> 0.117167586135   ,  \"σηlogτS\" -> 0.000047458198   ,  \"σηlogτN\" -> 0.130090926522   ,  \"σlogτ1\" -> 0.024427268103   ,  \"σlogτS\" -> 0.000080353339   ,  \"σlogτN\" -> 0.013579690528   ,  \"σητ1\" -> 0.002257953787   ,  \"σητS \" -> 0.000000860297   ,  \"σητN\" -> 0.000024921021    |>   , \n\"IDS0635_220612_RAW_cal__sam_\" ->   <|    \"ζ\" -> 0.000000000000   ,  \"τ1\" -> 0.000000000000   ,  \"τS\" -> 0.000000000000   ,  \"τN\" -> 0.000000000000   ,  \"τC\" -> 0.000000000000   ,  \"κ0\" -> 0.000000000000   ,  \"mm1\" -> 0.000000000000   ,  \"mm2\" -> 0.000000000000   ,  \"mm3\" -> 0.000000000000   ,  \"T\" -> 1.120000000000   ,  \"B\" -> 10.000000000000   ,  \"θ\" -> 90.000000000000   ,  \"Reoff\" -> 0.000000000000   ,  \"Imoff\" -> 0.000000000000   ,  \"στ1\" -> 0.000000000000   ,  \"στS\" -> 0.000000000000   ,  \"στN\" -> 0.000000000000   ,  \"τ11 \" -> 0.000000000000   ,  \"τ12\" -> 0.000000000000   ,  \"τ22\" -> 0.000000000000   ,  \"τN1\" -> 0.000000000000   ,  \"τN2\" -> 0.000000000000   ,  \"σηlogτ1 \" -> 0.000000000000   ,  \"σηlogτS\" -> 0.000000000000   ,  \"σηlogτN\" -> 0.000000000000   ,  \"σlogτ1\" -> 0.000000000000   ,  \"σlogτS\" -> 0.000000000000   ,  \"σlogτN\" -> 0.000000000000   ,  \"σητ1\" -> 0.000000000000   ,  \"σητS \" -> 0.000000000000   ,  \"σητN\" -> 0.000000000000    |>   , \n\"IDS0636_220612_RAW_cal__ref_\" ->   <|    \"ζ\" -> 0.017149890612   ,  \"τ1\" -> 0.022569079306   ,  \"τS\" -> 0.013897839626   ,  \"τN\" -> 0.000042116682   ,  \"τC\" -> 0.002942632523   ,  \"κ0\" -> 0.000000012622   ,  \"mm1\" -> 0.000041165605   ,  \"mm2\" -> 0.016909717626   ,  \"mm3\" -> 0.022739853632   ,  \"T\" -> 1.900000000000   ,  \"B\" -> 10.000000000000   ,  \"θ\" -> 90.000000000000   ,  \"Reoff\" -> 0.000000000000   ,  \"Imoff\" -> 0.000000000000   ,  \"στ1\" -> 0.001616870383   ,  \"στS\" -> 0.000000714504   ,  \"στN\" -> 0.000001915578   ,  \"τ11 \" -> 0.000000000000   ,  \"τ12\" -> 0.000000000000   ,  \"τ22\" -> 0.000000000000   ,  \"τN1\" -> 0.000000000000   ,  \"τN2\" -> 0.000000000000   ,  \"σηlogτ1 \" -> 0.096802089984   ,  \"σηlogτS\" -> 0.000006983072   ,  \"σηlogτN\" -> 0.125439998859   ,  \"σlogτ1\" -> 0.071640954450   ,  \"σlogτS\" -> 0.000051411167   ,  \"σlogτN\" -> 0.045482634513   ,  \"σητ1\" -> 0.002184734046   ,  \"σητS \" -> 0.000000097050   ,  \"σητN\" -> 0.000005283117    |>   , \n\"IDS0636_220612_RAW_cal__sam_\" ->   <|    \"ζ\" -> 0.000000000000   ,  \"τ1\" -> 0.000000000000   ,  \"τS\" -> 0.000000000000   ,  \"τN\" -> 0.000000000000   ,  \"τC\" -> 0.000000000000   ,  \"κ0\" -> 0.000000000000   ,  \"mm1\" -> 0.000000000000   ,  \"mm2\" -> 0.000000000000   ,  \"mm3\" -> 0.000000000000   ,  \"T\" -> 1.900000000000   ,  \"B\" -> 10.000000000000   ,  \"θ\" -> 90.000000000000   ,  \"Reoff\" -> 0.000000000000   ,  \"Imoff\" -> 0.000000000000   ,  \"στ1\" -> 0.000000000000   ,  \"στS\" -> 0.000000000000   ,  \"στN\" -> 0.000000000000   ,  \"τ11 \" -> 0.000000000000   ,  \"τ12\" -> 0.000000000000   ,  \"τ22\" -> 0.000000000000   ,  \"τN1\" -> 0.000000000000   ,  \"τN2\" -> 0.000000000000   ,  \"σηlogτ1 \" -> 0.000000000000   ,  \"σηlogτS\" -> 0.000000000000   ,  \"σηlogτN\" -> 0.000000000000   ,  \"σlogτ1\" -> 0.000000000000   ,  \"σlogτS\" -> 0.000000000000   ,  \"σlogτN\" -> 0.000000000000   ,  \"σητ1\" -> 0.000000000000   ,  \"σητS \" -> 0.000000000000   ,  \"σητN\" -> 0.000000000000    |>   , \n\"IDS0637_220612_RAW_cal__ref_\" ->   <|    \"ζ\" -> 0.017770105668   ,  \"τ1\" -> 0.021549186615   ,  \"τS\" -> 0.009965620739   
